vi "checkcomplete.vi"(8 "error in":errorcluster) -> (0 "error out":errorcluster)   [LabVIEW 2019]
uses:
  _ctrl/init-r-stop.ctl
  Glob_Ref.vi
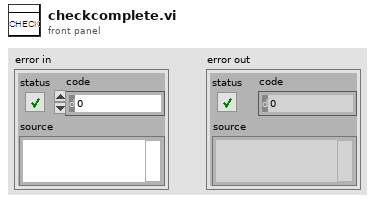
[diagram p1: front panel]
types:
  T1 = typedef "init-r-stop.ctl" = enum16{"ini", "read", "stop"}
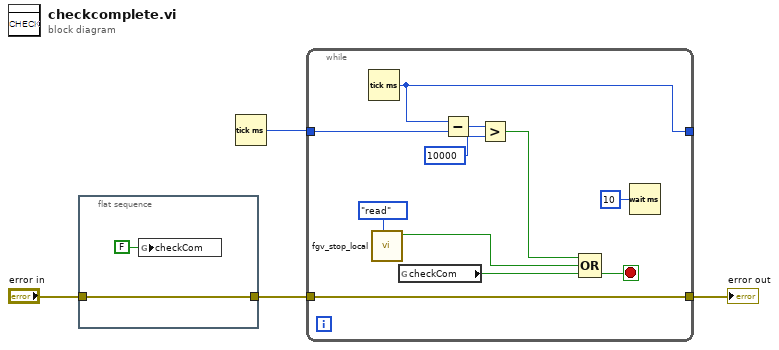
[diagram p0: block diagram]
diagram:
  n1 = flat-sequence {
    tunnel: [w5] -> w4
    tunnel: "error in" -> [w5]
    frame #0 {
      n2 = global write "Glob_Ref.vi" "checkCom"(FALSE ("checkCom")) -> ()
    }
  }
  n3 = Tick Count (ms)() -> (millisecond timer value=w1:u32)
  n4 = while {
    tunnel: w4 -> [w14]
    tunnel: [w14] -> w2
    tunnel: w1 -> [w12]
    tunnel: [w13] -> _
    stop <- w15 stop-if-true
    n5 = Tick Count (ms)() -> (millisecond timer value=w13:u32)
    n6 = call "fgv_stop_local.vi"("cmd"=init-r-stop."read") -> ("stop"=w7:bool)  [unwired: 10 in]
    n7 = global read "Glob_Ref.vi" "checkCom"() -> (w16:bool)
    n8 = Subtract(x=w13, y=w12) -> (x-y=w11:u32)
    n9 = Greater?(x=w11, y=u32 10000) -> (0:w9:bool)
    n10 = Compound Arithmetic op=OR(w9, w7, w16) -> (w15:bool)
    n11 = Wait (ms)(milliseconds to wait=u32 10) -> ()  [unwired: 1 out]
  }
  "error out" <- w2
